vi "Get Boolean Value.vi"(6 "Default Value":bool, 8 "error in (no error)":errorcluster, 10 "Name":string, 11 "Test Recipe in":refnum<class "Test Recipe.lvclass">) -> (0 "error out":errorcluster, 2 "Value":bool, 3 "Test Recipe out":refnum<class "Test Recipe.lvclass">)   [LabVIEW 2015]
uses:
  Test Recipe.lvclass
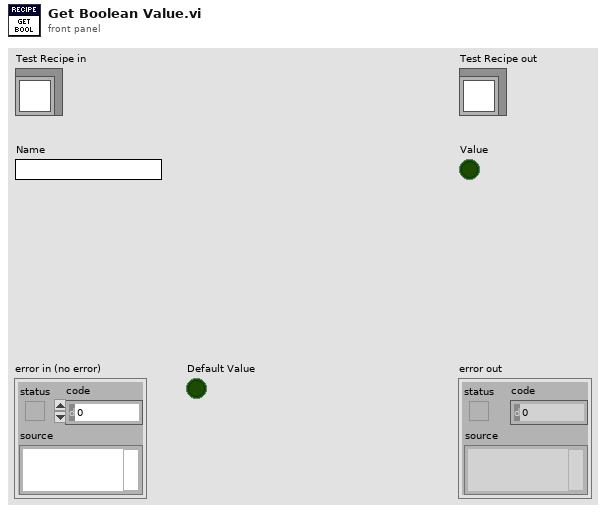
[diagram p1: front panel]
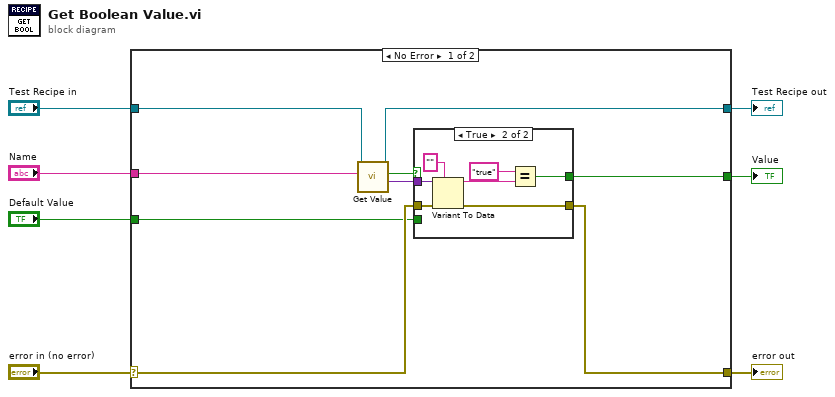
[diagram p0: block diagram]
diagram:
  n1 = case shown="No Error" "error in (no error)" {
    selector: "error in (no error)" -> [w11 w27]
    tunnel: [w10 w27] -> w6
    tunnel: [w15 w26] -> w4
    tunnel: "Test Recipe in" -> [w16 w26]
    tunnel: "Name" -> [w14 _]
    tunnel: [w12 _] -> w2
    tunnel: "Default Value" -> [w8 _]
    frame No Error {
      n2 = call-dynamic "Get Value.vi"("Key"=w14, "Registry in"=w16) -> ("Value"=w13:variant, "found?"=w9:bool, "Registry out"=w15:refnum<class "Test Recipe.lvclass">)  [unwired: 6 in, 1 out]
      n3 = case shown="True" w9 {
        tunnel: w13 -> [_ w25]
        tunnel: [w17 w19] -> w12
        tunnel: w11 -> [w18 w24]
        tunnel: [w18 w23] -> w10
        tunnel: w8 -> [w17 _]
        frame False {
        }
        frame True {
          n4 = Variant To Data(error in=w24, type="", Variant=w25) -> (data=w21:string, error out=w23:errorcluster)
          n5 = Equal?(x="true", y=w21) -> (x = y?=w19:bool)
        }
      }
    }
    frame Error {
    }
  }
  "error out" <- w6
  "Test Recipe out" <- w4
  "Value" <- w2
